vi "SaveFaultDetectionsToTDMS.vi"(8 "error in (no error)":errorcluster, 10 "Fault detections":T1, 11 "Refnum in":refnum<k34>) -> (0 "error out":errorcluster, 3 "tdms file out":refnum<k34>)   [LabVIEW 2019]
uses:
  MobileAnalyzer/mainVIs/analyzeAccelerationDataVIs/calculateFaultIndicatorsVIs/FaultDetections.ctl
  MobileAnalyzer/mainVIs/analyzeAccelerationDataVIs/calculateFaultIndicatorsVIs/ParameterFaultDetection.ctl
  MobileAnalyzer/mainVIs/analyzeAccelerationDataVIs/calculateFaultIndicatorsVIs/FaultParameter.ctl
  MobileAnalyzer/mainVIs/analyzeAccelerationDataVIs/calculateFaultIndicatorsVIs/FrequencyFaultDetection.ctl
  MobileAnalyzer/mainVIs/analyzeAccelerationDataVIs/calculateFaultIndicatorsVIs/OrdersFaultDetection.ctl
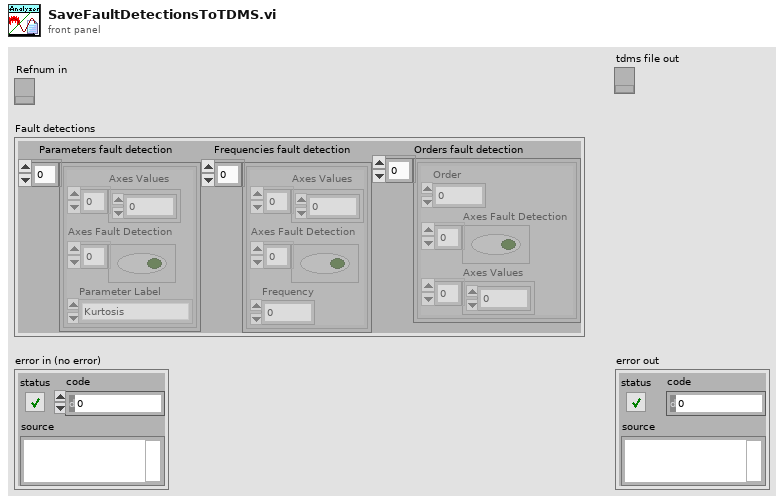
[diagram p1: front panel]
types:
  T1 = typedef "FaultDetections.ctl" = cluster{"Parameters fault detection":T2[], "Frequencies fault detection":T4[], "Orders fault detection":T5[]}
  T2 = typedef "ParameterFaultDetection.ctl" = cluster{"Axes Values":dbl[], "Axes Fault Detection":bool[], "Parameter Label":T3}
  T3 = typedef "FaultParameter.ctl" = enum16{"Kurtosis", "RMS", "Crest factor"}
  T4 = typedef "FrequencyFaultDetection.ctl" = cluster{"Axes Values":dbl[], "Axes Fault Detection":bool[], "Frequency":dbl}
  T5 = typedef "OrdersFaultDetection.ctl" = cluster{"Order":dbl, "Axes Fault Detection":bool[], "Axes Values":dbl[]}
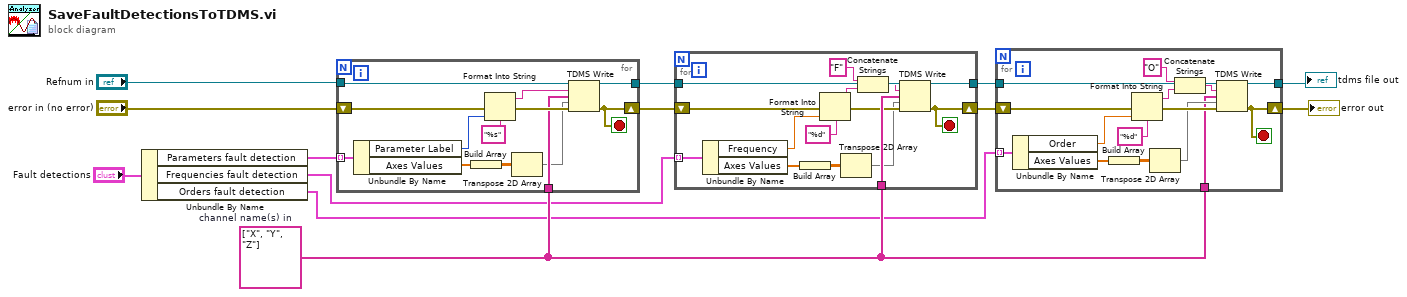
[diagram p0: block diagram]
diagram:
  w12 = string[] ["X", "Y", "Z"]  # channel name(s) in
  n1 = Unbundle By Name("Fault detections") -> ("Parameters fault detection"=w5:T2[], "Frequencies fault detection"=w7:T4[], "Orders fault detection"=w11:T5[])
  n2 = for {
    tunnel: w5 -> [w26] mode=indexing
    shift-right: [w19] -> w6
    shift-left: "error in (no error)" -> [w25]
    tunnel: "Refnum in" -> [w22]
    tunnel: w12 -> [w18]
    tunnel: [w17] -> w8
    stop <- w19 stop-if-true
    n3 = Unbundle By Name(w26) -> ("Parameter Label"=w21:T3, "Axes Values"=w16:dbl[])
    n4 = Build Array(w16) -> (w15:dbl[][])
    n5 = Format Into String(format string="%s", error in=w25, w21) -> (resulting string=w20:string, error out=w23:errorcluster)  [unwired: 1 in]
    n6 = Transpose 2D Array(2D array=w15) -> (transposed array=w14:dbl[][])
    n7 = TDMS Write(0:w22, 5:w20, 7:w18, 9:w14, 11:w23) -> (4:w17:refnum<k34>, 15:w19:errorcluster)  [unwired: 1 in, 2 out]
  }
  n8 = for {
    tunnel: w7 -> [w41] mode=indexing
    shift-right: [w39] -> w9
    shift-left: w6 -> [w37]
    tunnel: w8 -> [w40]
    tunnel: w12 -> [w38]
    tunnel: [w30] -> w13
    stop <- w39 stop-if-true
    n9 = Unbundle By Name(w41) -> ("Frequency"=w36:dbl, "Axes Values"=w32:dbl[])
    n10 = Build Array(w32) -> (w33:dbl[][])
    n11 = Format Into String(format string="%d", error in=w37, w36) -> (resulting string=w28:string, error out=w34:errorcluster)  [unwired: 1 in]
    n12 = Transpose 2D Array(2D array=w33) -> (transposed array=w31:dbl[][])
    n13 = Concatenate Strings("F" ("format string"), w28) -> (w29:string)
    n14 = TDMS Write(0:w40, 5:w29, 7:w38, 9:w31, 11:w34) -> (4:w30:refnum<k34>, 15:w39:errorcluster)  [unwired: 1 in, 2 out]
  }
  n15 = for {
    shift-right: [w47] -> w10
    shift-left: w9 -> [w55]
    tunnel: w11 -> [w56] mode=indexing
    tunnel: w12 -> [w48]
    tunnel: w13 -> [w46]
    tunnel: [w42] -> w1
    stop <- w47 stop-if-true
    n16 = Unbundle By Name(w56) -> ("Order"=w52:dbl, "Axes Values"=w50:dbl[])
    n17 = Build Array(w50) -> (w51:dbl[][])
    n18 = Format Into String(format string="%d", error in=w55, w52) -> (resulting string=w44:string, error out=w54:errorcluster)  [unwired: 1 in]
    n19 = Transpose 2D Array(2D array=w51) -> (transposed array=w49:dbl[][])
    n20 = Concatenate Strings("O" ("format string"), w44) -> (w45:string)
    n21 = TDMS Write(0:w46, 5:w45, 7:w48, 9:w49, 11:w54) -> (4:w42:refnum<k34>, 15:w47:errorcluster)  [unwired: 1 in, 2 out]
  }
  "error out" <- w10
  "tdms file out" <- w1
